vi "Test - Moving Objects Source.vi"() -> ()   [LabVIEW 2019]
doc: "This VI is used as a test VI by the Moving Objects example VIs."
panel:
  in  "Move Me - Numeric":dbl
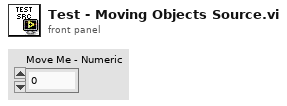
[diagram p1: front panel]
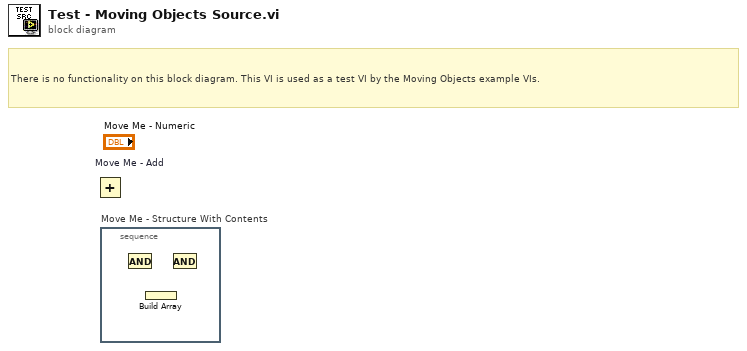
[diagram p0: block diagram]
diagram:
  # "There is no functionality on this block diagram. This VI is used as a test VI by the Moving Objects example VIs."
  n1 = Add "Move Me - Add"() -> ()  [unwired: 2 in, 1 out]
  n2 = stacked-sequence "Move Me - Structure With Contents" {
    frame #0 {
      n3 = And() -> ()  [unwired: 2 in, 1 out]
      n4 = Build Array() -> ()  [unwired: 1 in, 1 out]
      n5 = And() -> ()  [unwired: 2 in, 1 out]
    }
  }
